vi "installer_create.vi"(6 "distribution_folder":path, 8 "error in (no error)":errorcluster, 11 "build_specifications":T1) -> (0 "error out":errorcluster)   [LabVIEW 2015, in "lv-builder-default.lvlib"]
uses:
  lv-builder-default.lvlib
  lv-build/public/_controls/build_specification.ctl
  lv-build/public/_controls/build_type.ctl
  <userlib>/antonio-alexander/lv-bin-7zip/public/api/v1/_controls/config_include.ctl
  <userlib>/antonio-alexander/lv-bin-7zip/public/api/v1/_controls/config_value.ctl
  <userlib>/antonio-alexander/lv-bin-7zip/public/api/v1/advanced/make_installer_exe_custom.vi
  <userlib>/antonio-alexander/lv-bin-7zip/public/api/v1/v1.lvlib
  lv-build/lv-build.lvlib
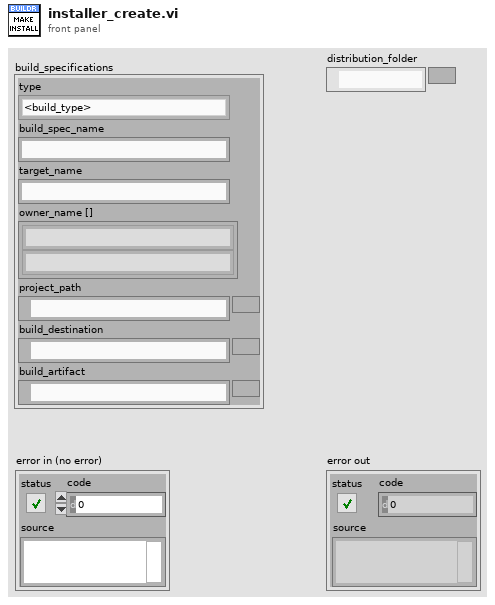
[diagram p1: front panel]
types:
  T1 = typedef "lv-build.lvlib/build_specification.ctl" = cluster{"type":T2, "build_spec_name":string, "target_name":string, "owner_name []":string[], "project_path":path, "build_destination":path, "build_artifact":path}
  T2 = typedef "lv-build.lvlib/build_type.ctl" = enum16{"<build_type>", "application_pc", "application_rt", "installer", "llb", "lvlibp", "zip", "fpga", "<null>"}
  T3 = typedef "lv-bin-7zip.lvlib/v1.lvlib/config_value.ctl" = cluster{"title":string, "begin_prompt":string, "run_program":string, "directory":string, "execute_file":string, "execute_parameters":string, "progress":bool}
  T4 = typedef "lv-bin-7zip.lvlib/v1.lvlib/config_include.ctl" = cluster{"title":bool, "begin_prompt":bool, "progress":bool, "run_program":bool, "directory":bool, "execute_file":bool, "execute_parameters":bool}
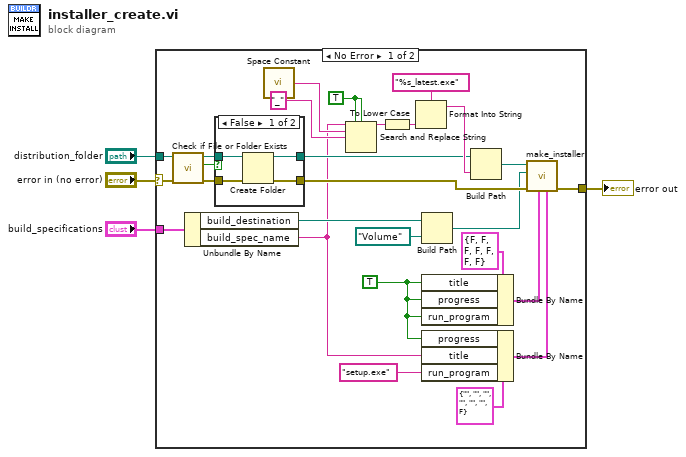
[diagram p0: block diagram]
diagram:
  n1 = case shown="No Error" "error in (no error)" {
    selector: "error in (no error)" -> [w13 w38]
    tunnel: "build_specifications" -> [w30 _]
    tunnel: [w25 w38] -> w4
    tunnel: "distribution_folder" -> [w6 _]
    frame No Error {
      w18 = TRUE ("replace all? (F)")
      w7 = TRUE ("title")
      n2 = call <vilib>:"Check if File or Folder Exists.vi"("error in (no error)"=w13, "path"=w6) -> ("error out"=w12:errorcluster, "file or folder exists?"=w9:bool, "dup path"=w11:path)  [unwired: 7 in]
      n3 = Unbundle By Name(w30) -> ("build_destination"=w24:path, "build_spec_name"=w5:string)
      n4 = case shown="False" w9 {
        tunnel: w12 -> [w35 w36]
        tunnel: w11 -> [w34 w37]
        tunnel: [w33 w37] -> w10
        tunnel: [w32 w36] -> w31
        frame False {
          n5 = Create Folder(path (use dialog)=w34, error in=w35) -> (created path=w33:path, error out=w32:errorcluster)  [unwired: 1 in, 1 out]
        }
        frame True {
        }
      }
      n6 = call <vilib>:"Space Constant.vi"() -> ("String"=w15:string)
      n7 = Search and Replace String(replace all?=w18, case sensitive?=w18, input string=w5, search string=w15, replace string="_" ("search string")) -> (result string=w16:string)  [unwired: 3 in, 3 out]
      n8 = To Lower Case(string=w16) -> (all lower case string=w17:string)
      n9 = Format Into String(format string="%s_latest.exe", w17) -> (resulting string=w28:string)  [unwired: 2 in, 1 out]
      n10 = Build Path(base path=w24, name or relative path=path "Volume") -> (appended path=w26:path)
      n11 = Bundle By Name(cluster=T4 {"title"=FALSE, "begin_prompt"=FALSE, "progress"=FALSE, "run_program"=FALSE, "directory"=FALSE, "execute_file"=FALSE, "execute_parameters"=FALSE} ("config_include"), "title"=w7, "progress"=w7, "run_program"=w7) -> (w21:T4)
      n12 = Bundle By Name(cluster=T3 {"title"="", "begin_prompt"="", "run_program"="", "directory"="", "execute_file"="", "execute_parameters"="", "progress"=FALSE} ("config_value"), "progress"=w7, "title"=w5, "run_program"="setup.exe") -> (w20:T3)
      n13 = Build Path(base path=w10, name or relative path=w28) -> (appended path=w27:path)
      n14 = call-poly <userlib>:"make_installer.vi"("config_value"=w20, "config_include"=w21, "error in (no error)"=w31, "installer_directory"=w26, "setup_filename in"=w27) -> ("error out"=w25:errorcluster)  [unwired: 5 in, 1 out]
    }
    frame Error {
    }
  }
  "error out" <- w4
